vi "Parse_MetadataJSONFILE.vi"(8 "error in (no error)":errorcluster, 11 "File or Folder Path":path) -> (0 "error out":errorcluster, 1 "file or folder exists?":bool, 2 "output cluster":T17 {"Sorted scan parameters"."?"."Rate" format="%.2f"; "Sorted scan parameters"."?"."Step" format="%#_6p"; "Sorted scan parameters"."?"."End" format="%#_6p"; "Sorted scan parameters"."?"."Start" format="%#_6p"})   [LabVIEW 2016]
uses:
  <userlib>/LevyLab/Lockin-Multichannel/Typedefs/Function-enum.ctl
  <userlib>/LevyLab/Lockin-Multichannel/Typedefs/Function-array.ctl
  <userlib>/LevyLab/Lockin-Multichannel/Typedefs/AO_phi-array.ctl
  <userlib>/LevyLab/Lockin-Multichannel/Typedefs/AO_f-array.ctl
  <userlib>/LevyLab/Lockin-Multichannel/Typedefs/AO_DC-array.ctl
  <userlib>/LevyLab/Lockin-Multichannel/Typedefs/AO_Amp-array.ctl
  <userlib>/LevyLab/Lockin-Multichannel/Typedefs/AO-cluster.ctl
  levylab_expt_transport/src/SMOs/SweepControl/Typedefs/Enum - PostAction.ctl
  levylab_expt_transport/src/SMOs/SweepControl/SweepControl.lvclass
  levylab_expt_transport/src/SMOs/SweepControl/Typedefs/PostAction.ctl
  levylab_expt_transport/src/SMOs/SweepControl/Typedefs/Enum - Action.ctl
  levylab_expt_transport/src/SMOs/SweepControl/Typedefs/Enum - Priority.ctl
  levylab_expt_transport/src/SMOs/SweepControl/Typedefs/Cluster - ScanControl.ctl
  levylab_expt_transport/src/SMOs/SweepControl/Typedefs/ScanControl.ctl
  levylab_expt_transport/src/subVI/SweepMetadata.ctl
  <vilib>/addons/_JKI.lib/Serialization/JSON/JKI JSON Serialization.lvlib
  levylab_expt_transport/src/subVI/SweepMetadataV2.ctl
  levylab_expt_transport/src/SMOs/SweepControl/Typedefs/ScanParamters.ctl
  levylab_expt_transport/src/SMOs/SweepControl/Typedefs/Cluster - ScanParamters.ctl
panel:
  out "Sweep Metadata Cluster":T1 {"Channels: AO"."AO f (Hz)" min=0.001 max=10000.0; "Channels: AO"."AO DC (V)" format="%#_6p"; "Channels: AO"."AO amp (V)" format="%#_6p"}
  out "# Of Sweep Pts. Fast to Slow":i16[](array[numeric])
  out "Sorted scan parameters":cluster{T15}[](array[cluster])=[{[{"Start"=0.14, "End"=-0.060000000000000005, "Step"=-0.060000000000000005, "Rate"=0.0, "wait (ms)"=10000, "address"="\nscaledVsg1=", "Channel"=2}]}, {[{"Start"=0.14, "End"=-0.060000000000000005, "Step"=-0.060000000000000005, "Rate"=0.0, "wait (ms)"=10000, "address"="\nscaledVsg1=", "Channel"=2}]}, {[{"Start"=0.14, "End"=-0.060000000000000005, "Step"=-0.060000000000000005, "Rate"=0.0, "wait (ms)"=10000, "address"="\nscaledVsg1=", "Channel"=2}, {"Start"=0.14, "End"=-0.060000000000000005, "Step"=-0.060000000000000005, "Rate"=0.0, "wait (ms)"=10000, "address"="\nscaledVsg1=", "Channel"=3}]}] {"?"."Rate" format="%.2f"; "?"."Step" format="%#_6p"; "?"."End" format="%#_6p"; "?"."Start" format="%#_6p"}
  out "Sorted scan control":cluster{T11}[](array[cluster])=[{[{"Priority"=enum."Priority 0", "Scan name"=enum."DSA_Vsg2"}]}, {[{"Priority"=enum."Priority 1", "Scan name"=enum."DSA_Vamp"}]}, {[{"Priority"=enum."Priority 2", "Scan name"=enum."DSA_Vsg1"}, {"Priority"=enum."Priority 2", "Scan name"=enum."DSA_Vsg3"}]}]
  # "1st = # of lowest number priority = highest priority"
  # "0"
  # "1"
  # "2"
  # "3"
  # "4"
  # "5"
  # "6"
  # "7"
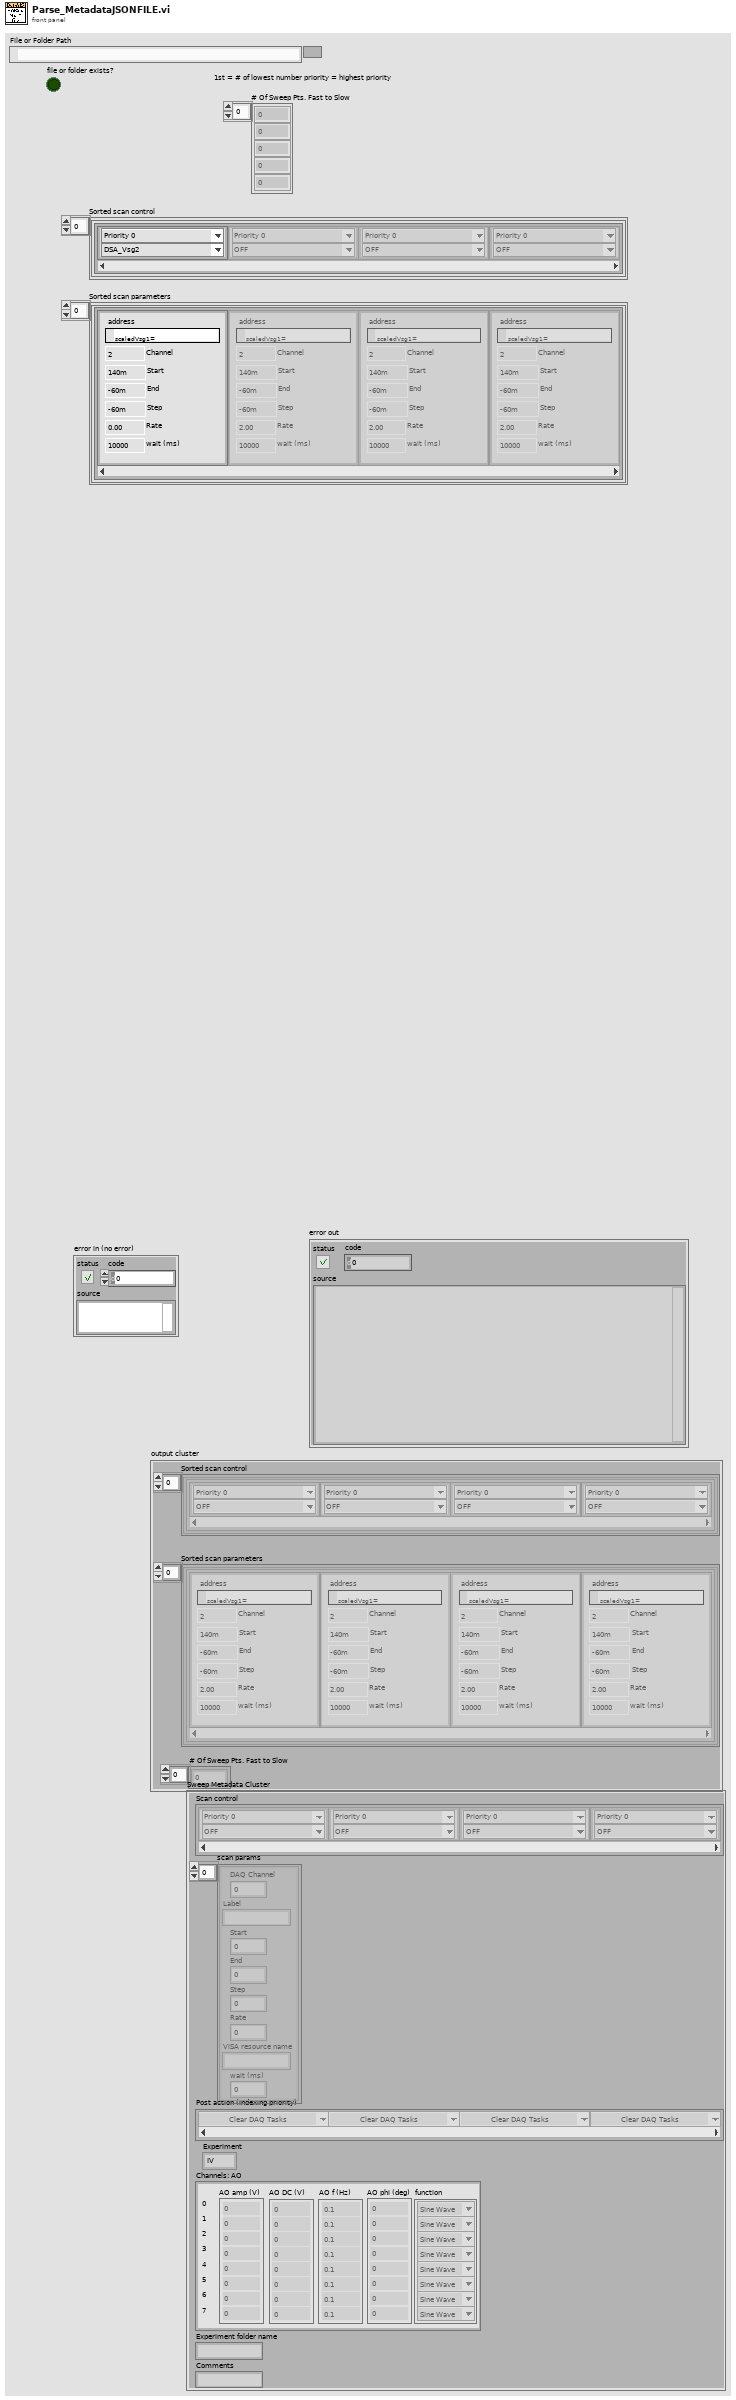
[diagram p1: front panel]
types:
  T1 = typedef "SweepMetadataV2.ctl" = cluster{"Experiment":enum16{"IV", "lockin_time", "Lockin_Vsg"}, "Experiment folder name":string, "Comments":string, "Channels: AO":T2, "Post action (indexing priority)":T9, "Scan control":T11, "scan params":cluster{"DAQ Channel":i32, "Label":string, "Start":dbl, "End":dbl, "Step":dbl, "Rate":dbl, "VISA resource name":string, "wait (ms)":u32}[]}
  T2 = typedef "AO-cluster.ctl" = cluster{"AO amp (V)":T3, "AO DC (V)":T4, "AO f (Hz)":T5, "AO phi (deg)":T6, "function":T7}
  T3 = typedef "AO_Amp-array.ctl" = dbl[]
  T4 = typedef "AO_DC-array.ctl" = dbl[]
  T5 = typedef "AO_f-array.ctl" = dbl[]
  T6 = typedef "AO_phi-array.ctl" = dbl[]
  T7 = typedef "Function-array.ctl" = T8[]
  T8 = typedef "Function-enum.ctl" = enum16{"Sine Wave", "Triangle Wave", "Square Wave", "Sawtooth Wave"}
  T9 = typedef "SweepControl.lvclass/PostAction.ctl" = T10[]
  T10 = typedef "SweepControl.lvclass/Enum - PostAction.ctl" = enum16{"Clear DAQ Tasks", "Check Temperature", "Wait", "Do Nothing"}
  T11 = typedef "SweepControl.lvclass/ScanControl.ctl" = T12[]
  T12 = typedef "SweepControl.lvclass/Cluster - ScanControl.ctl" = cluster{"Priority":T13, "Scan name":T14}
  T13 = typedef "SweepControl.lvclass/Enum - Priority.ctl" = enum16{"Priority 0", "Priority 1", "Priority 2", "Priority 3", "Priority 4", "Priority 5"}
  T14 = typedef "SweepControl.lvclass/Enum - Action.ctl" = enum16{"OFF", "DSA_Vamp", "DSA_freq", "DSA_Vsg1", "DSA_Vsg2", "DSA_Vsg3", "DAQ_Vbg", "B_Field", "Humidity", "Temp", "MW_freq1", "MW_freq2", "MW_amplitude1", "MW_amplitude2"}
  T15 = typedef "SweepControl.lvclass/ScanParamters.ctl" = T16[]
  T16 = typedef "SweepControl.lvclass/Cluster - ScanParamters.ctl" = cluster{"Start":dbl, "End":dbl, "Step":dbl, "Rate":dbl, "wait (ms)":u32, "address":refnum<visa-resource-name>, "Channel":i32}
  T17 = cluster{"Sorted scan control":cluster{T11}[], "Sorted scan parameters":cluster{T15}[], "# Of Sweep Pts. Fast to Slow":i16[]}
  T18 = typedef "SweepMetadata.ctl" = cluster{"Scan control":T11, "Scan Parameters":cluster{"DAQ Channel":i32, "Label":string, "Start":dbl, "End":dbl, "Step":dbl, "Rate":dbl, "VISA resource name":string, "wait (ms)":u32}[], "Post action (indexing priority)":T9, "Experiment":enum16{"IV", "lockin_time", "Lockin_Vsg"}, "Channels: AO":T2, "Experiment folder name":string, "Comments":string}
  T19 = cluster{"Experiment":enum16{"IV", "lockin_time", "Lockin_Vsg"}, "Experiment folder name":string, "Comments":string, "Channels: AO":T2, "Post action (indexing priority)":T9, "Scan control":T11, "scan params":cluster{"DAQ Channel":i32, "Label":string, "Start":dbl, "End":dbl, "Step":dbl, "Rate":dbl, "wait (ms)":u32, "visa resource name":string}[]}
  T20 = cluster{"Sorted scan control":cluster{T11}[], "Sorted scan parameters":cluster{T15}[], i16[]}
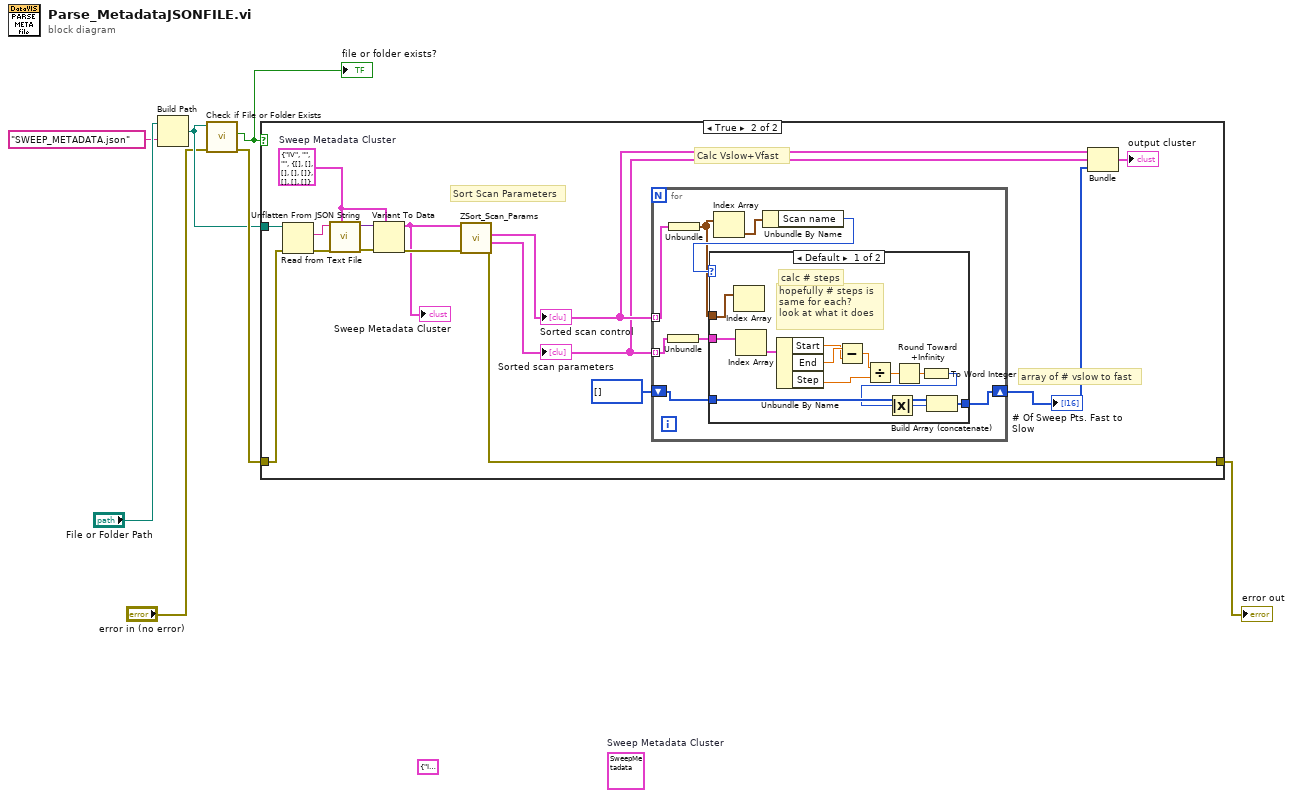
[diagram p0: block diagram]
diagram:
  (unwired) T18 {"Scan control"=[], "Scan Parameters"=[], "Post action (indexing priority)"=[], "Experiment"=enum."IV", "Channels: AO"={"AO amp (V)"=[], "AO DC (V)"=[], "AO f (Hz)"=[], "AO phi (deg)"=[], "function"=[]}, "Experiment folder name"="", "Comments"=""}  # Sweep Metadata Cluster
  (unwired) T19 {"Experiment"=enum."IV", "Experiment folder name"="", "Comments"="", "Channels: AO"={"AO amp (V)"=[], "AO DC (V)"=[], "AO f (Hz)"=[], "AO phi (deg)"=[], "function"=[]}, "Post action (indexing priority)"=[], "Scan control"=[], "scan params"=[]} ("output cluster 2")
  n1 = Build Path(base path="File or Folder Path", name or relative path="SWEEP_METADATA.json") -> (appended path=w5:path)
  n2 = call <vilib>:"Check if File or Folder Exists.vi"("error in (no error)"="error in (no error)", "path"=w5) -> ("error out"=w6:errorcluster, "file or folder exists?"=w4:bool)  [unwired: 7 in, 1 out]
  "file or folder exists?" <- w4
  n3 = case shown="True" w4 {
    tunnel: w5 -> [_ w22]
    tunnel: w6 -> [w8 w18]
    tunnel: [w8 w16] -> w2
    frame False {
    }
    frame True {
      w10 = T1 {"Experiment"=enum."IV", "Experiment folder name"="", "Comments"="", "Channels: AO"={"AO amp (V)"=[], "AO DC (V)"=[], "AO f (Hz)"=[], "AO phi (deg)"=[], "function"=[]}, "Post action (indexing priority)"=[], "Scan control"=[], "scan params"=[]}  # Sweep Metadata Cluster
      # "array of # vslow to fast"
      # "Calc Vslow+Vfast"
      # "Sort Scan Parameters"
      n4 = Read from Text File(file (use dialog)=w22, error in=w18) -> (text=w21:string, error out=w19:errorcluster)  [unwired: 2 in, 2 out]
      n5 = call <vilib>:"Unflatten From JSON String.vi"("Type and Defaults"=w10, "error in (no error)"=w19, "JSON String"=w21) -> ("error out"=w20:errorcluster, "Variant"=w23:variant)  [unwired: 7 in]
      n6 = Variant To Data(error in=w20, type=w10, Variant=w23) -> (data=w9:T1, error out=w17:errorcluster)
      "Sweep Metadata Cluster" <- w9
      n7 = call "ZSort_Scan_Params.vi"("error in (no error)"=w17, "Sweep Metadata Cluster"=w9) -> ("error out"=w16:errorcluster, "Sorted scan parameters"=w13:cluster{T15}[], "Sorted scan control"=w14:cluster{T11}[])  [unwired: 7 in]
      "Sorted scan control" <- w14
      "Sorted scan parameters" <- w13
      n8 = for {
        tunnel: w14 -> [w31] mode=indexing
        tunnel: w13 -> [w27] mode=indexing
        shift-right: [w24] -> w12
        shift-left: i16[] [] -> [w25]
        n9 = Unbundle(w27) -> (w26:T15)
        n10 = Unbundle(w31) -> (w28:T11)
        n11 = Index Array(array=w28) -> (element=w30:T12)  [unwired: 1 in]
        n12 = Unbundle By Name(w30) -> ("Scan name"=w29:T14)
        n13 = case shown="Default" w29 {
          tunnel: w28 -> [w44 _]
          tunnel: w26 -> [w43 _]
          tunnel: w25 -> [w37 w45]
          tunnel: [w36 w45] -> w24
          frame Default {
            # "hopefully # steps is\nsame for each?\nlook at what it does"
            # "calc # steps"
            n14 = Index Array(array=w44) -> ()  [unwired: 1 in, 1 out]
            n15 = Index Array(array=w43) -> (element=w42:T16)  [unwired: 1 in]
            n16 = Unbundle By Name(w42) -> ("Start"=w40:dbl, "End"=w41:dbl, "Step"=w38:dbl)
            n17 = Subtract(x=w41, y=w40) -> (x-y=w39:dbl)
            n18 = Divide(x=w39, y=w38) -> (x/y=w35:dbl)
            n19 = Round Toward +Infinity(x=w35) -> (ceil(x): smallest int >= x=w34:dbl)
            n20 = To Word Integer(number=w34) -> (16bit integer=w33:i16)
            n21 = Absolute Value(x=w33) -> (abs(x)=w32:i16)
            n22 = Build Array (concatenate)(w37, w32) -> (w36:i16[])
          }
          frame "OFF" {
            # "Ignore this one"
          }
        }
      }
      "# Of Sweep Pts. Fast to Slow" <- w12
      n23 = Bundle("Sorted scan control"=w14, "Sorted scan parameters"=w13, w12) -> (→"output cluster":T20)  [unwired: 1 in]
    }
  }
  "error out" <- w2
